vi "detector_acquire_generic_data.vi"(8 "error in (no error)":errorcluster, 11 "tt20 in":refnum<class "tt20.lvclass">) -> (0 "error out":errorcluster, 2 "image_data":T1, 3 "tt20 out":refnum<class "tt20.lvclass">)   [LabVIEW 2015, in "tt20.lvclass"]
uses:
  tt20.lvclass
  Experiment/experiment_panel/2d_scan/detector_data_tdef.ctl
  tt20.lvclass/tt20.ctl
  C:/Users/MX-Microscope/Documents/LabVIEW Data/lvoop_campus_2018/Detector_Class/Swabian/time_tagger_vis/TTCSharp32.dll
  time_tagger_vis/TTCSharp32.dll
  <vilib>/Analysis/baseanly.llb/Mean (DBL).vi
  <vilib>/Analysis/NI_AALBase.lvlib
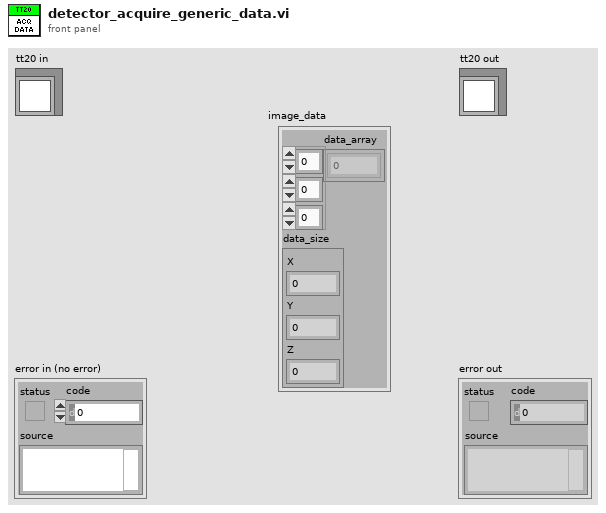
[diagram p1: front panel]
types:
  T1 = typedef "detector_data_tdef.ctl" = cluster{"data_array":dbl[][][], "data_size":cluster{"X":i32, "Y":i32, "Z":i32}}
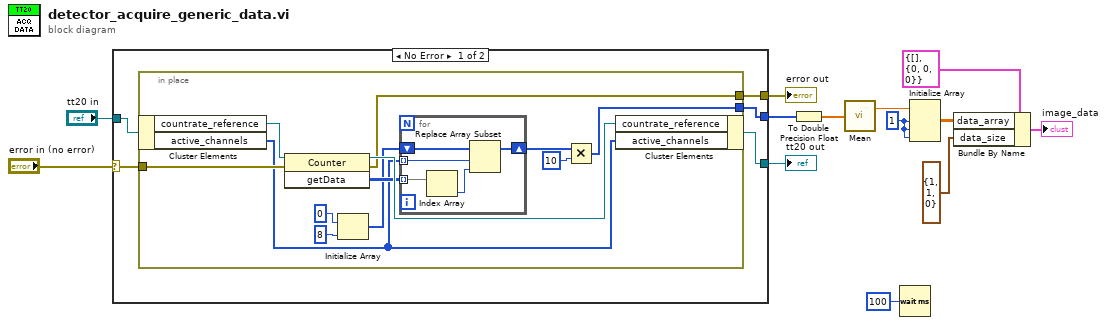
[diagram p0: block diagram]
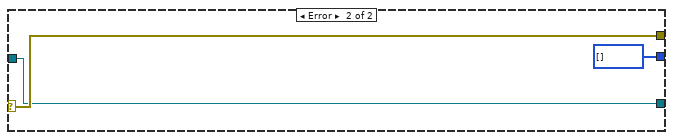
[diagram p2: hidden frame]
diagram:
  w13 = 1 ("dimension size")
  n1 = case shown="No Error" "error in (no error)" {
    selector: "error in (no error)" -> [w17 w38]
    tunnel: "tt20 in" -> [w18 w36]
    tunnel: [w16 w36] -> w6
    tunnel: [w14 i32[] [] ("getData")] -> w3
    tunnel: [w15 w38] -> w7
    frame No Error {
      n2 = in-place {
        in-place-border: w17 -> [w28]
        in-place-border: [w27] -> w15
        in-place-border: [w25] -> w14
        n3 = in-place-cluster #1(w18) -> ("countrate_reference"=w30:refnum<k24>, "active_channels"=w19:u32[])
        n4 = invoke class="Counter" method="getData"(reference=w30, error in=w28) -> (reference out=w29:refnum<k24>, error out=w27:errorcluster, "getData"=w24:i32[][])  [unwired: 1 in]
        n5 = Initialize Array(0, 8 ("dimension size")) -> (w21:i32[])
        n6 = for {
          tunnel: w24 -> [w35] mode=indexing
          tunnel: w19 -> [w34] mode=indexing
          shift-right: [w31] -> w20
          shift-left: w21 -> [w33]
          n7 = Index Array(array=w35) -> (element=w32:i32)  [unwired: 1 in]
          n8 = Replace Array Subset(array=w33, new element=w32, index=w34) -> (w31:i32[])
        }
        n9 = Multiply(x=w20, y=10) -> (x*y=w25:i32[])
        n10 = in-place-cluster #1("countrate_reference"=w29, "active_channels"=w19) -> (w16:refnum<class "tt20.lvclass">)
      }
    }
    frame Error {
    }
  }
  "error out" <- w7
  "tt20 out" <- w6
  n11 = To Double Precision Float(number=w3) -> (double precision float=w2:dbl[])
  n12 = call-poly <vilib>:"Mean.vi"("X"=w2) -> ("mean"=w12:dbl)  [unwired: 1 out]
  n13 = Wait (ms)(milliseconds to wait=u32 100) -> ()  [unwired: 1 out]
  n14 = Initialize Array(w12, w13, w13, w13) -> (w10:dbl[][][])
  n15 = Bundle By Name(cluster=T1 {"data_array"=[], "data_size"={"X"=0, "Y"=0, "Z"=0}} ("image_data"), "data_array"=w10, "data_size"=cluster{"X":i32, "Y":i32, "Z":i32} {"X"=1, "Y"=1, "Z"=0}) -> (→"image_data":T1)
